vi "test_Add Command_Use SysDef With Only Custom Device.vi"(8 "error in (no error)":errorcluster, 11 "TestCase in":refnum<class "Instrument Addon Scripting API Messages Unit Tests.lvclass">) -> (0 "error out":errorcluster, 3 "TestCase out":refnum<class "Instrument Addon Scripting API Messages Unit Tests.lvclass">)   [LabVIEW 2018, in "Instrument Addon Scripting API Messages Unit Tests.lvclass"]
uses:
  Instrument Addon Scripting API Messages Unit Tests.lvclass
  Addon/Addon Shared/Types/FG Control.ctl
  APIs/Scripting API/TypeDefs/Settings.ctl
  <vilib>/NI Veristand/Custom Device API/Custom Device Item Ref.ctl
  APIs/Scripting API/TypeDefs/Padding.ctl
  Addon/Addon Shared/Types/Command Parameters.ctl
  Addon/Addon Shared/Types/Linked Channel Cluster.ctl
  Addon/Addon Shared/SubVIs/Constants.vi
  <vilib>/NI/NI VeriStand Advanced SysDef API/_SubVIs/SysDef.Search.GUID.vi
  <vilib>/NI Veristand/Custom Device API/NI VeriStand - Get Item Property.vi
  <vilib>/NI Veristand/Custom Device API/Get Item Property (String).vi
  <vilib>/NI Veristand/Custom Device API/Get Item Property (String Array).vi
  <vilib>/NI Veristand/Custom Device API/Get Item Property (Boolean).vi
  <vilib>/NI Veristand/Custom Device API/Get Item Property (U32).vi
  <vilib>/NI Veristand/Custom Device API/NI VeriStand - Set Item Property.vi
  <vilib>/NI Veristand/Custom Device API/Set Item Property (String).vi
  <vilib>/NI Veristand/Custom Device API/Set Item Property (String Array).vi
  <vilib>/NI Veristand/Custom Device API/Set Item Property (Boolean).vi
  <vilib>/NI Veristand/Custom Device API/Set Item Property (U32).vi
  <vilib>/addons/_JKI Toolkits/VI Tester/TestCase.llb/TestCase.lvclass
  Instrument Addon Scripting API Test Assets/Instrument Addon Scripting API Test Assets.lvclass
  APIs/Scripting API/Instrument Addon Scripting API.lvlib
  Addon/Addon Shared/Instrument Addon Shared.lvlib
  <vilib>/NI/NI VeriStand Advanced SysDef API/SysDef API/Advanced System Definition.lvlib
  <vilib>/NI VeriStand/Custom Device API/Custom Device API.lvlib
  C:/Program Files (x86)/National Instruments/LabVIEW 2018/vi.lib/addons/_JKI Toolkits/VI Tester/TestCase.llb/TestCase.lvclass
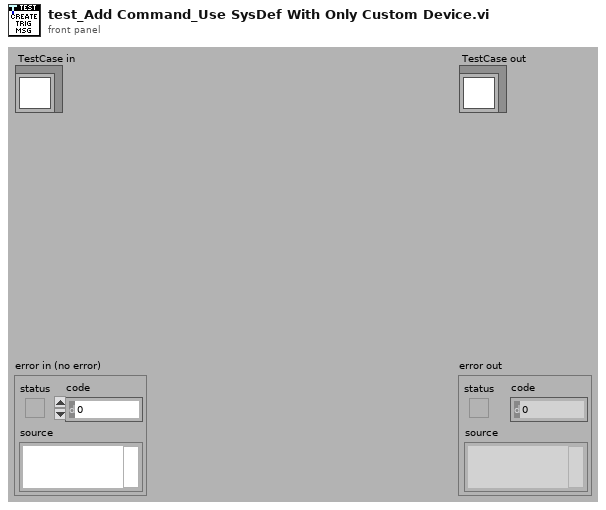
[diagram p1: front panel]
types:
  T1 = typedef "Custom Device API.lvlib/Custom Device Item Ref.ctl" = u64
  T2 = cluster{"Variable Name":string, "Channel Ref in":T1}[]
  T3 = typedef "Instrument Addon Scripting API.lvlib/Settings.ctl" = cluster{"Command Format":string, "Linked Channels":cluster{"Variable Name":string, "Channel Ref in":T1}[], "Pad":bool, "Padding":T4}
  T4 = typedef "Instrument Addon Scripting API.lvlib/Padding.ctl" = cluster{"Pad Value":u8, "Length":u32}
  T5 = typedef "Instrument Addon Shared.lvlib/FG Control.ctl" = enum16{"Get", "Set"}
  T6 = typedef "Instrument Addon Shared.lvlib/Command Parameters.ctl" = cluster{"Command":string, "Linked Channels":T7[], "Pad":bool, "Length":u32, "Pad Value":u8}
  T7 = typedef "Instrument Addon Shared.lvlib/Linked Channel Cluster.ctl" = cluster{"Variable Name":string, "GUID":string}
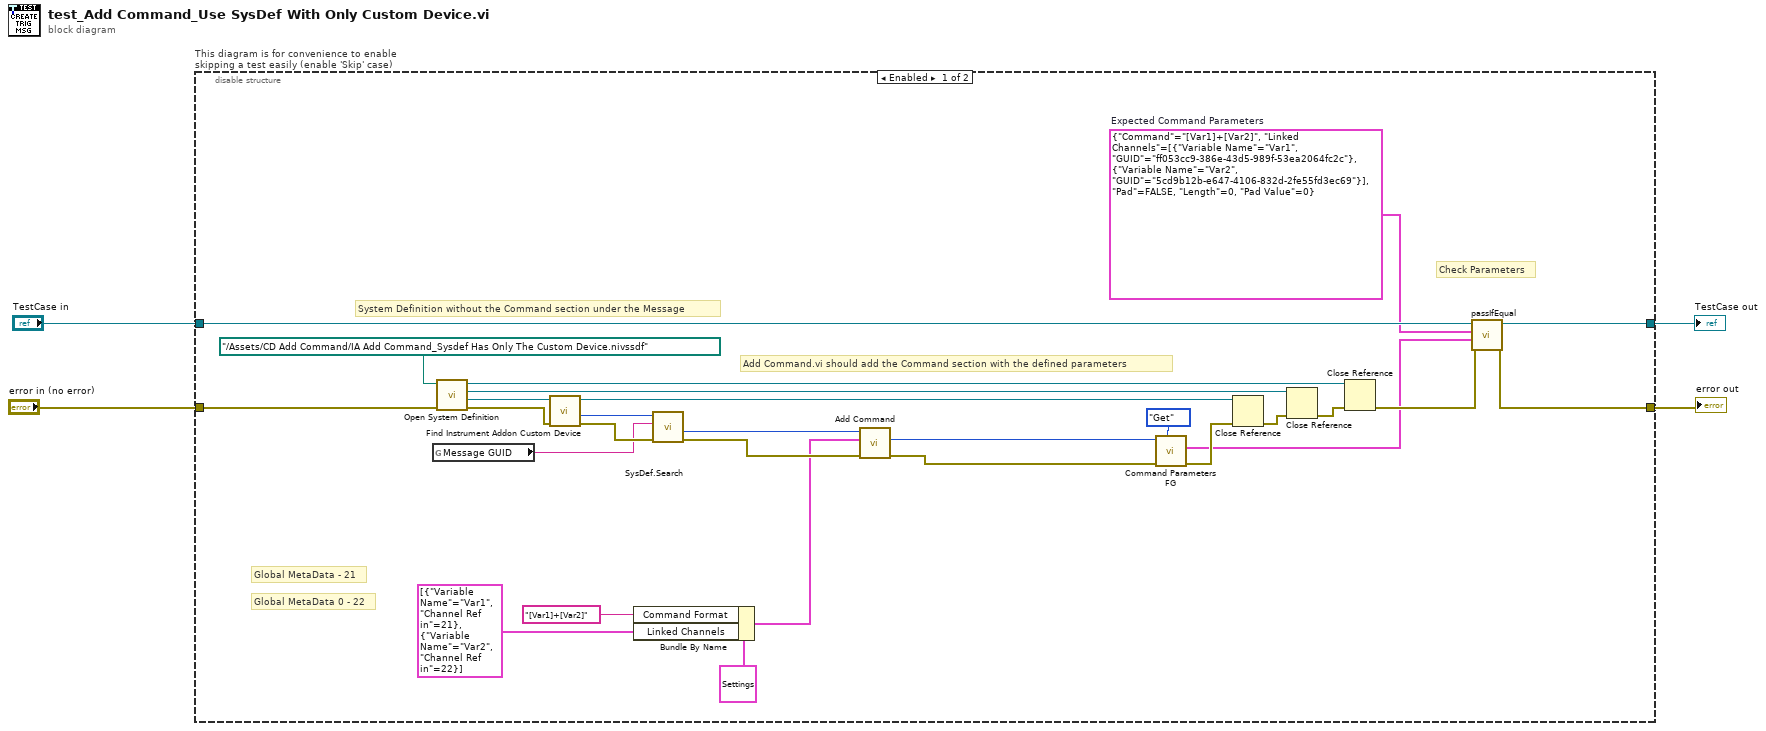
[diagram p0: block diagram]
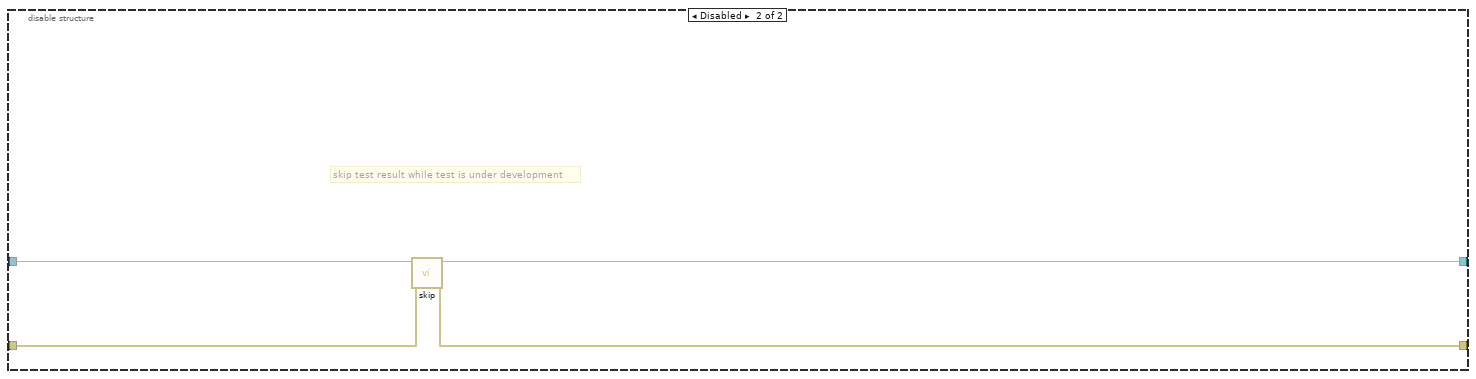
[diagram p2: hidden frame]
diagram:
  n1 = disable-structure "This diagram is for convenience to enable skipping a test easily (enable 'Skip' case)" shown="Enabled" {
    disable-tunnel: "TestCase in" -> [w29 w36]
    disable-tunnel: [w25 w34] -> w1
    disable-tunnel: [w26 w35] -> w3
    disable-tunnel: "error in (no error)" -> [w31 w33]
    frame Enabled {
      w5 = T6 {"Command"="[Var1]+[Var2]", "Linked Channels"=[{"Variable Name"="Var1", "GUID"="ff053cc9-386e-43d5-989f-53ea2064fc2c"}, {"Variable Name"="Var2", "GUID"="5cd9b12b-e647-4106-832d-2fe55fd3ec69"}], "Pad"=FALSE, "Length"=0, "Pad Value"=0}  # Expected Command Parameters
      # "Add Command.vi should add the Command section with the defined parameters"
      # "System Definition without the Command section under the Message"
      # "Check Parameters"
      # "Global MetaData 0 - 22"
      # "Global MetaData - 21"
      n2 = global read "Constants.vi" "Message GUID"() -> (w14:string)
      n3 = call "Open System Definition.vi"("error in (no error)"=w31, "System Definition File"=path "../Assets/CD Add Command/IA Add Command_Sysdef Has Only The Custom Device.nivssdf" ("SDF file")) -> ("error out"=w16:errorcluster, "Target Refnum"=w17:refnum<k24>, "Root Refnum"=w30:refnum<k24>, "System Definition Refnum"=w22:refnum<k24>)  [unwired: 6 in]
      n4 = call "Find Instrument Addon Custom Device.vi"("error in"=w16, "target in"=w17) -> ("error out"=w15:errorcluster, "NodeID"=w7:u64, "target out"=w8:refnum<k24>)  [unwired: 7 in]
      n5 = Bundle By Name(cluster=T3 {"Command Format"="[Var1]+[Var2]", "Linked Channels"=[{"Variable Name"="Var1", "Channel Ref in"=32}, {"Variable Name"="Var2", "Channel Ref in"=33}], "Pad"=FALSE, "Padding"={"Pad Value"=0, "Length"=0}} ("Settings"), "Command Format"="[Var1]+[Var2]", "Linked Channels"=T2 [{"Variable Name"="Var1", "Channel Ref in"=21}, {"Variable Name"="Var2", "Channel Ref in"=22}]) -> (w10:T3)
      n6 = call-poly <vilib>:"SysDef.Search.vi"("error in (no error)"=w15, "GUID"=w14, "nodeID"=w7) -> ("error out"=w12:errorcluster, "Value out"=w13:u64)  [unwired: 5 in, 2 out]
      n7 = call "Add Command.vi"("error in (no error)"=w12, "Settings"=w10, "Message Refnum In"=w13) -> ("error out"=w21:errorcluster, "Command Refnum"=w20:T1)  [unwired: 6 in, 1 out]
      n8 = call "Command Parameters FG.vi"("Action"=FG_Control."Get", "error in (no error)"=w21, "Item Ref in"=w20) -> ("error out"=w19:errorcluster, "Command Parameters"=w18:T6)  [unwired: 6 in, 1 out]
      n9 = Close Reference(reference=w8, error in (no error)=w19) -> (error out=w24:errorcluster)
      n10 = Close Reference(reference=w30, error in (no error)=w24) -> (error out=w28:errorcluster)
      n11 = Close Reference(reference=w22, error in (no error)=w28) -> (error out=w27:errorcluster)
      n12 = call-dynamic "passIfEqual.vi"("error in (no error)"=w27, "y"=w18, "x"=w5, "TestCase in"=w29) -> ("error out"=w26:errorcluster, "TestCase out"=w25:refnum<class "Instrument Addon Scripting API Messages Unit Tests.lvclass">)  [unwired: 6 in]
    }
    frame Disabled {
      # "skip test result while test is under development"
      n13 = call <vilib>:"skip.vi"("error in (no error)"=w33, "TestCase in"=w36) -> ("error out"=w35:errorcluster, "TestCase out"=w34:refnum<class "Instrument Addon Scripting API Messages Unit Tests.lvclass">)  [unwired: 8 in]
    }
  }
  "error out" <- w3
  "TestCase out" <- w1
